vi "401_Read_Audit_Data.vi"(8 "error in (no error)":errorcluster, 11 "Refnum in":T1) -> (0 "error out":errorcluster, 3 "Refnum out":T1, 6 "Data_Table":string[][](array[string]))   [LabVIEW 2015]
uses:
  <vilib>/addons/database/Connection.llb/Conn ObjectReference.ctl
  <vilib>/addons/database/Connection.llb/DB Tools Open Connec (String).vi
  <vilib>/addons/database/NI_Database_API.lvlib
panel:
  # "Outputs"
  # "Inputs"
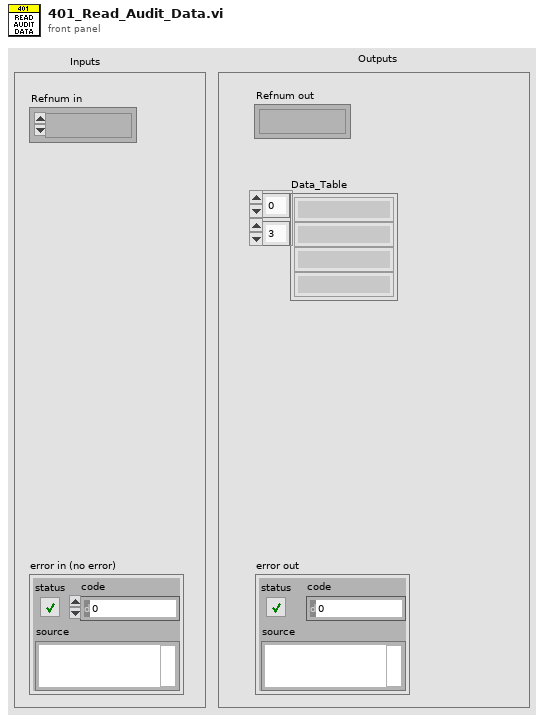
[diagram p1: front panel]
types:
  T1 = typedef "NI_Database_API.lvlib/Conn ObjectReference.ctl" = refnum<k1>
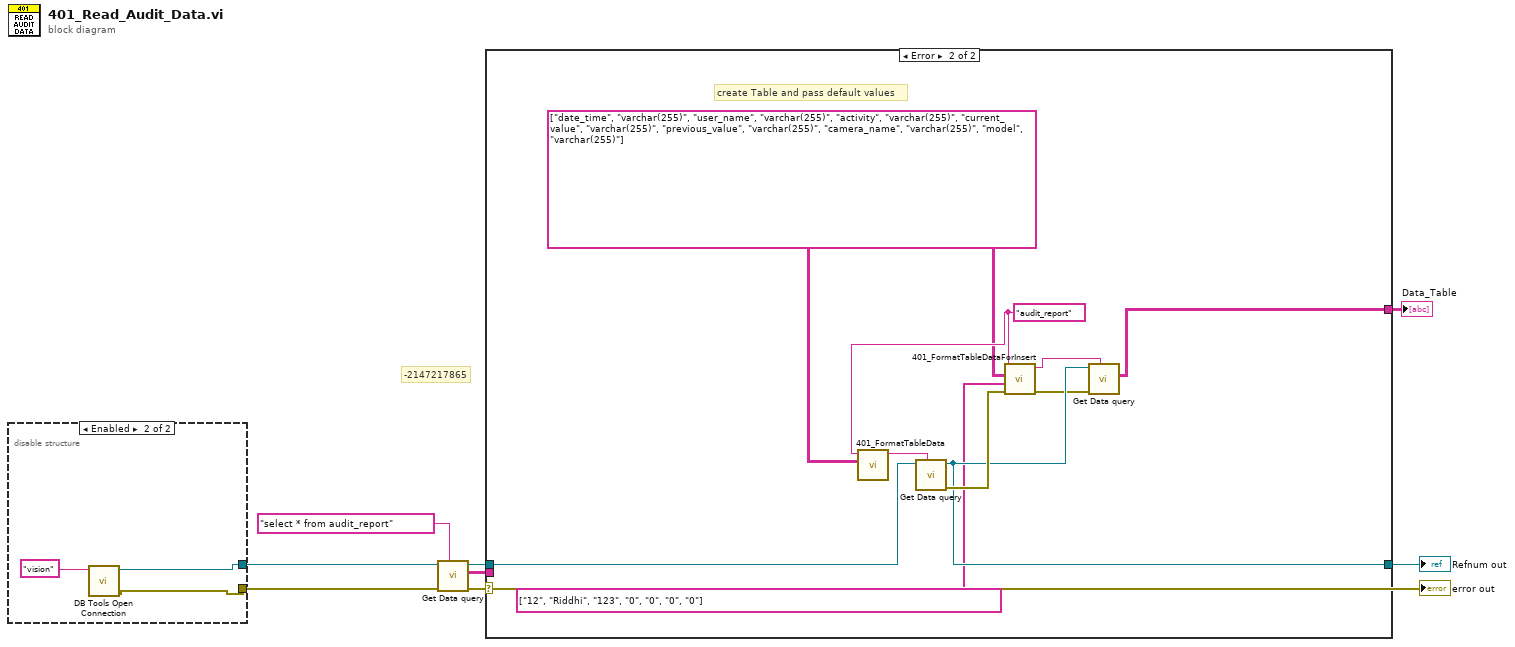
[diagram p0: block diagram]
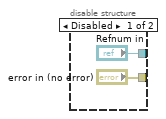
[diagram p3: hidden frame]
diagram:
  # "-2147217865"
  n1 = disable-structure shown="Enabled" {
    disable-tunnel: ["error in (no error)" w11] -> w6
    disable-tunnel: ["Refnum in" w12] -> w1
    frame Disabled {
    }
    frame Enabled {
      n2 = call-poly <vilib>:"DB Tools Open Connection.vi"("connection information"="vision" ("userID")) -> ("error out"=w11:errorcluster, "connection reference"=w12:T1)  [unwired: 7 in]
    }
  }
  n3 = call "Get Data query.vi"("SQL query"="select * from audit_report", "error in"=w6, "connection reference"=w1) -> ("error Out"=w5:errorcluster, "Data_Table"=w8:string[][], "connection reference"=w4:T1)  [unwired: 6 in]
  "error out" <- w5
  n4 = case shown="Error" w5 {
    tunnel: [w14 w16] -> w2
    tunnel: w8 -> [w14 _]
    tunnel: w4 -> [w15 w24]
    tunnel: [w15 w21] -> w3
    frame No Error {
    }
    frame Error {
      w17 = string[][] [["date_time", "varchar(255)"], ["user_name", "varchar(255)"], ["activity", "varchar(255)"], ["current_value", "varchar(255)"], ["previous_value", "varchar(255)"], ["camera_name", "varchar(255)"], ["model", "varchar(255)"]] ("ColoumnNames+DataType")
      w23 = "audit_report" ("Table_Name")
      # "create Table and pass default values"
      n5 = call "401_FormatTableData.vi"("ColoumnNames+DataType"=w17, "Table_Name"=w23) -> ("Query"=w25:string)  [unwired: 9 in]
      n6 = call "Get Data query.vi"("SQL query"=w25, "connection reference"=w24) -> ("error Out"=w22:errorcluster, "connection reference"=w21:T1)  [unwired: 7 in, 1 out]
      n7 = call "401_FormatTableDataForInsert.vi"("Error In"=w22, "Values"=string[] ["12", "Riddhi", "123", "0", "0", "0", "0"], "ColoumnNames+DataType"=w17, "Table_Name"=w23) -> ("ErrorOut"=w20:errorcluster, "Query"=w19:string)  [unwired: 6 in]
      n8 = call "Get Data query.vi"("SQL query"=w19, "error in"=w20, "connection reference"=w21) -> ("Data_Table"=w16:string[][])  [unwired: 6 in, 2 out]
    }
  }
  "Refnum out" <- w3
  "Data_Table" <- w2
